vi "RegisterForDiagPackets.vi"(7 "error in (no error)":errorcluster, 9 "refresh interval (default)":i32, 10 "Controller in":refnum<k24>) -> (0 "error out":errorcluster, 1 "Event Metadata":T1, 2 "Event Registration Refnum":refnum<event-registration>, 3 "Controller out":refnum<k24>)   [LabVIEW 2016, in "Aerotech VIs.lvlib"]
uses:
  Aerotech VIs.lvlib
  C:/Program Files (x86)/Aerotech/A3200/LabVIEW/2010/Bin/Aerotech.A3200.dll
  ControllerDiagPacket.ctl
  AxisDiagPacket.ctl
  C:/Program Files (x86)/Aerotech/A3200/LabVIEW/2010/Bin/Aerotech.A3200.LabVIEW.dll
panel:
  in  "ControllerDiagPacket":T2
  in  ".Net Event":refnum<k27>
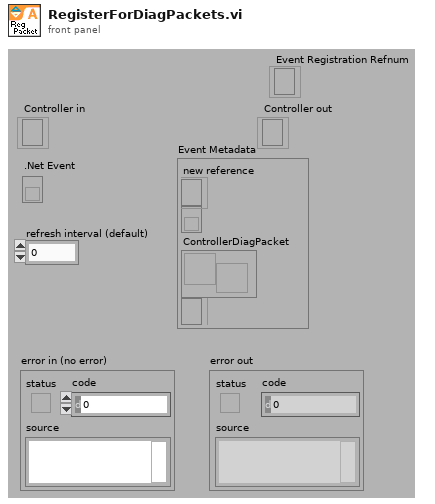
[diagram p1: front panel]
types:
  T1 = cluster{"new reference":refnum<k24>, "Event Callback":refnum<k27>, "ControllerDiagPacket":refnum<user-event>, "Event Registration Refnum":refnum<event-registration>}
  T2 = typedef "Aerotech VIs.lvlib/ControllerDiagPacket.ctl" = cluster{"Number of Diag Packets":i32, "Axes":T3[], "error":errorcluster}
  T3 = typedef "Aerotech VIs.lvlib/AxisDiagPacket.ctl" = cluster{"Axis Name":string, "Analog Input 0":dbl, "Analog Input 1":dbl, "Axis Fault (num)":i32, "Axis Fault (str)":string, "Axis Fault (bits)":cluster{"AmplifierFault":bool, "AmplifierTemperatureFault":bool, "CcwEndOfTravelLimitFault":bool, "CcwSoftwareLimitFault":bool, "CommunicationLostFault":bool, "CwEndOfTravelLimitFault":bool, "CwSoftwareLimitFault":bool, "EmergencyStopFault":bool, "EncoderFault":bool, "ExternalFault":bool, "FeedbackScalingFault":bool, "GantryMisalignFault ":bool, "HallSensorFault":bool, "InPositionTimeoutFault":bool, "MarkerSearchFault":bool, "MaxVelocityCommandFault":bool, "MotorTemperatureFault":bool, "None":bool, "OverCurrentFault":bool, "PositionErrorFault":bool, "PositionFeedbackFault":bool, "PowerSupplyFault":bool, "ProbeInputFault":bool, "SafeZoneFault":bool, "VelocityErrorFault":bool, "VelocityFeedbackFault":bool, "VoltageClampFault":bool}, "Axis Status (num)":i32, "Axis Status (str)":string, "Axis Status (bits)":cluster{"BacklashActive":bool, "CalibrationEnabled1D":bool, "CalibrationEnabled2D":bool, "CommandValid":bool, "DriveAbortPending":bool, "DrivePending":bool, "Enabling":bool, "GainMappingEnabled":bool, "GantryAligned":bool, "GantryRealigning":bool, "Homed":bool, "Homing":bool, "IFOVEnabled":bool, "JogGenerating":bool, "Jogging":bool, "JoystickControl":bool, "MasterSlaveControl":bool, "MotionBlocked":bool, "MotionClamped":bool, "MoveDone":bool, "None":bool, "NotVirtual":bool, "Profiling":bool, "Stability0":bool, "Stability1":bool, "TrajectoryFiltering":bool, "WaitDone":bool}, "Current Command":sgl, "Current Error":sgl, "Current Feedback":sgl, "Digital Inputs":i32, "Digital Outputs":i32, "Drive Status":i32, "Drive Status (str)":string, "Drive Status (bits)":cluster{"AccelerationPhase":bool, "AutofocusActive":bool, "BrakeOutput":bool, "CcwEndOfTravelLimitInput":bool, "CosineEncoderError":bool, "CurrentClamp":bool, "CwEndOfTravelLimitInput":bool, "DecelerationPhase":bool, "DualLoopActive":bool, "EmergencyStopInput":bool, "Enabled":bool, "EncoderClipping":bool, "GalvoCalibrationEnabled":bool, "GalvoPowerCorrection":bool, "HallAInput":bool, "HallBInput":bool, "HallCInput":bool, "HighResolutionMode":bool, "HomeLimitInput":bool, "InPosition":bool, "InPosition2":bool, "MarkerInput":bool, "MarkerLatch":bool, "MoveActive":bool, "NoMotorSupply":bool, "None":bool, "PowerLimiting":bool, "ProgrammingFlash":bool, "ProgrammingMXH":bool, "PSOHaltLatch":bool, "ServoControl":bool, "SineEncoderError":bool}, "Position Feedback Auxiliary":dbl, "Position Command":dbl, "Position Error":dbl, "Position Feedback":dbl, "Program Position Command":dbl, "Program Position Error":dbl, "Program Position Feedback":dbl, "Velocity Command":dbl, "Velocity Error":dbl, "Velocity Feedback":dbl}
  T4 = cluster{"new reference":refnum<k24>, refnum<k27>, "ControllerDiagPacket":refnum<user-event>, "Event Registration Refnum":refnum<event-registration>}
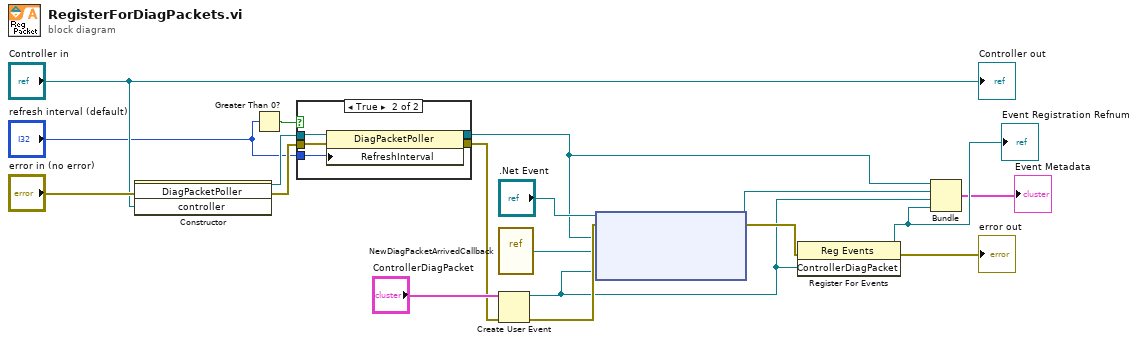
[diagram p0: block diagram]
diagram:
  n1 = constructor class="DiagPacketPoller"(error in="error in (no error)", "controller"="Controller in") -> (reference out=w8:refnum<k24>, error out=w7:errorcluster)  [unwired: 2 in, 2 out]
  n2 = Greater Than 0?(x="refresh interval (default)") -> (x > 0?=w4:bool)
  n3 = case shown="True" w4 {
    tunnel: "refresh interval (default)" -> [_ w25]
    tunnel: w8 -> [w20 w24]
    tunnel: w7 -> [w19 w23]
    tunnel: [w20 w22] -> w6
    tunnel: [w19 w21] -> w3
    frame False {
    }
    frame True {
      n4 = property class="DiagPacketPoller"(reference=w24, error in=w23, "RefreshInterval"=w25) -> (reference out=w22:refnum<k24>, error out=w21:errorcluster)
    }
  }
  n5 = vi-ref "NewDiagPacketArrivedCallback.vi"() -> ("vi reference"=w9:refnum<vi>)
  n6 = Create User Event(user event datatype="ControllerDiagPacket", error in=w3) -> (user event=w11:refnum<user-event>, error out=w14:errorcluster)
  n7 = node(".Net Event", w14, w6, w9, w11) -> (w10:refnum<k27>, w12:errorcluster)
  n8 = register-events(error in=w12, w11) -> (reference out=w2:refnum<event-registration>, error out=→"error out":errorcluster)  [unwired: 1 in]
  "Event Registration Refnum" <- w2
  n9 = Bundle("new reference"=w6, w10, "ControllerDiagPacket"=w11, "Event Registration Refnum"=w2) -> (→"Event Metadata":T4)  [unwired: 1 in]
  "Controller out" <- "Controller in"
